vi "ValueChangeSalirHMI.vi"(8 "error in (no error)":errorcluster) -> (0 "error out":errorcluster)   [LabVIEW 2018]
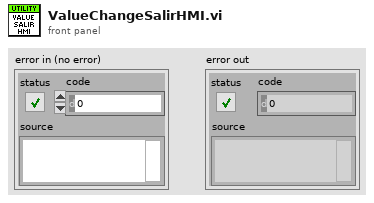
[diagram p1: front panel]
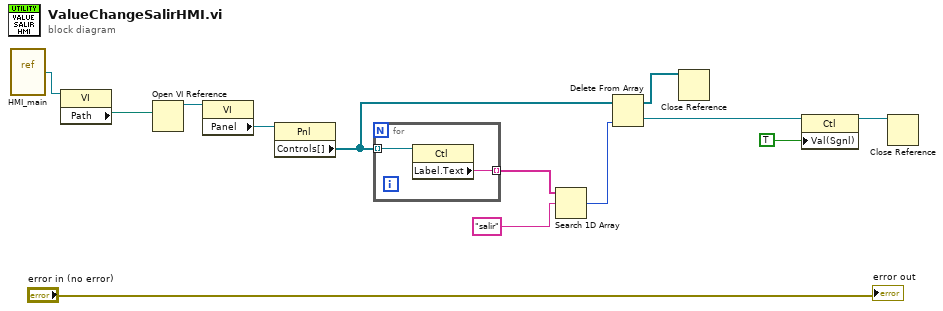
[diagram p0: block diagram]
diagram:
  n1 = vi-ref "HMI_main.vi"() -> (w11:refnum<vi>)
  n2 = property class="VI"(reference=w11) -> ("Path"=w12:path)  [unwired: 1 in, 2 out]
  n3 = Open VI Reference(vi path=w12) -> (vi reference=w9:refnum<vi>)  [unwired: 5 in, 1 out]
  n4 = property class="VI"(reference=w9) -> ("Panel"=w10:refnum<vi>)  [unwired: 1 in, 2 out]
  n5 = property class="Pnl"(reference=w10) -> ("Controls[]"=w6:refnum<vi>[])  [unwired: 1 in, 2 out]
  n6 = for {
    tunnel: w6 -> [w15] mode=indexing
    tunnel: [w14] -> w8 mode=indexing
    n7 = property class="Ctl"(reference=w15) -> ("Label.Text"=w14:string)  [unwired: 1 in, 2 out]
  }
  n8 = Search 1D Array(1D array=w8, element="salir" ("Nombre")) -> (index of element=w5:i32)  [unwired: 1 in]
  n9 = Delete From Array(array=w6, index=w5) -> (deleted portion=w3:refnum<vi>, array with subset deleted=w4:refnum<vi>[])  [unwired: 1 in]
  n10 = Close Reference(reference=w4) -> ()  [unwired: 1 in, 1 out]
  n11 = property class="Ctl"(reference=w3, "Val(Sgnl)"=TRUE) -> (reference out=w2:refnum<vi>)  [unwired: 1 in, 1 out]
  n12 = Close Reference(reference=w2) -> ()  [unwired: 1 in, 1 out]
  "error out" <- "error in (no error)"
